vi "Get Limit Voltage.vi"(8 "error in (no error)":errorcluster, 11 "hdl in":i32) -> (0 "error out":errorcluster, 2 "v limit":dbl, 3 "hdl out":i32)   [LabVIEW 2011, in "Thorlabs_MDT69xB.lvlib"]
doc: "Returns output voltage limit setting."
uses:
  <instrlib>/Thorlabs_MDT69xB/Thorlabs_MDT69xB.lvlib
  <instrlib>/Thorlabs_MDT69xB/Data/MDT_COMMAND_LIB_x64.dll
  <instrlib>/Thorlabs_MDT69xB/Data/MDT_COMMAND_LIB_win32.dll
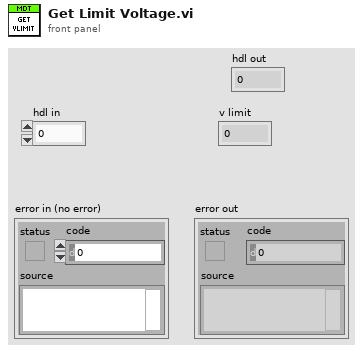
[diagram p1: front panel]
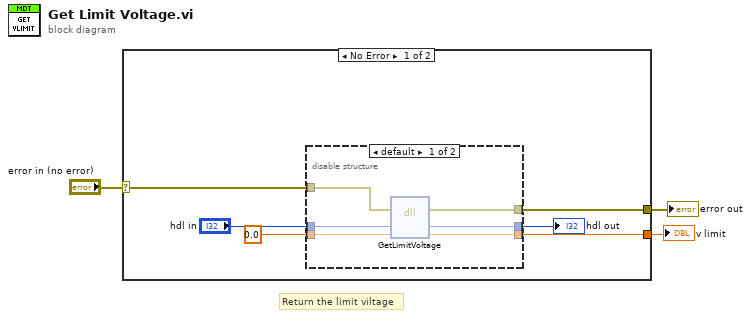
[diagram p0: block diagram]
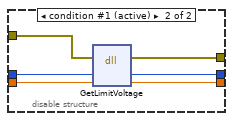
[diagram p2: hidden frame]
diagram:
  # "Return the limit viltage"
  n1 = case shown="No Error" "error in (no error)" {
    selector: "error in (no error)" -> [w8 w22]
    tunnel: [w7 w22] -> w2
    tunnel: [w5 _] -> w1
    frame No Error {
      n2 = disable-structure shown="default" {
        disable-tunnel: "hdl in" -> [w15 w21]
        disable-tunnel: w8 -> [w14 w20]
        disable-tunnel: [w13 w19] -> w7
        disable-tunnel: 0.0 ("voltage") -> [w12 w18]
        disable-tunnel: [w11 w17] -> w5
        disable-tunnel: [w10 w16] -> w4
        frame condition #0 {
          n3 = dll-call lib="E:/Program Files (x86)/National Instruments/LabVIEW 2011/instr.lib/Thorlabs_MDT69xB/Data/MDT_COMMAND_LIB_win32.dll" fn="GetLimitVoltage"(error in=w14, "hdl"=w15, "voltage"=w12) -> (error out=w13:errorcluster, "hdl"=w10:i32, "voltage"=w11:dbl)  [unwired: 3 in, 1 out]
        }
        frame condition #1 (active) {
          n4 = dll-call lib="C:/Program Files/National Instruments/LabVIEW 2011/instr.lib/Thorlabs_MDT69xB/Data/MDT_COMMAND_LIB_x64.dll" fn="GetLimitVoltage"(error in=w20, "hdl"=w21, "voltage"=w18) -> (error out=w19:errorcluster, "hdl"=w16:i32, "voltage"=w17:dbl)  [unwired: 3 in, 1 out]
        }
      }
      "hdl out" <- w4
    }
    frame Error {
    }
  }
  "error out" <- w2
  "v limit" <- w1
